vi "niFpgaScaledWinTemplate.vi"(0 "real data in":fxp<+/-,16,1>, 5 "imaginary data in":fxp<+/-,16,1>) -> (3 "data index":u16, 4 "real data out":fxp<+/-,18,2> format="%.17g", 6 "imaginary data out":fxp<+/-,18,2> format="%.17g")   [LabVIEW 2017]
uses:
  <vilib>/Platform/TimedLoop/XDataNode/timing_clust.ctl
  <vilib>/Platform/TimedLoop/XDataNode/nitl_modes.ctl
  <vilib>/Platform/TimedLoop/XDataNode/wakeup.ctl
  <vilib>/Platform/TimedLoop/XDataNode/XDataNode.xnode
  <vilib>/rvi/FXPMathLib/basic elements/FxpDiscreteDelay/XNode/nifxpmath_DiscreteDelay.xnode
  <vilib>/rvi/FXPMathLib/FxpMul/XNode/nifxpmath_Multiplier.xnode
  <vilib>/Platform/TimedLoop/XDataNode/XDNodeRunTimeDep.lvlib
  <vilib>/rvi/FXPMathLib/sim/FxpSim.dll
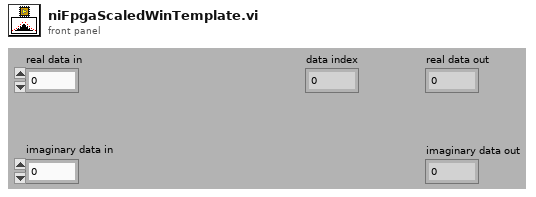
[diagram p1: front panel]
types:
  T1 = typedef "XDNodeRunTimeDep.lvlib/timing_clust.ctl" = cluster{"Expected End [f-1]":u64, "Actual End [f-1]":u64, "Finished Late? [f-1]":bool, "Expected End [i-1]":u64, "Actual End [i-1]":u64, "Finished Late? [i-1]":bool, "Expected Start [i]":u64, "Actual Start [i]":u64, "Expected Start [f]":u64, "Actual Start [f]":u64, "Source Name":string, "Structure Name":string, "Period":i64, "Deadline":i64, "Offset":i64, "Start":i64, "Priority":i32, "Timeout":i32, "Mode":T2, "Wakeup Reason":T3, "Error":errorcluster, "Source Type":string, "Secondary Source Type":string, "Global End Time":u64, "Global Start Time":u64, "Frame Duration":u64, "Iteration Duration":u64, "Assigned CPU":i32, "I/O Scan Engine Mode":u32}
  T2 = typedef "XDNodeRunTimeDep.lvlib/nitl_modes.ctl" = enum32{"No Change", "Process missed periods, maintain original phase", "Discard missed periods, maintain original phase", "Process missed periods, ignore original phase", "Discard missed periods, ignore original phase"}
  T3 = typedef "XDNodeRunTimeDep.lvlib/wakeup.ctl" = enum32{"Normal", "Aborted", "Asynchronous wakeup", "Timing source error", "Timed loop error", "Timeout"}
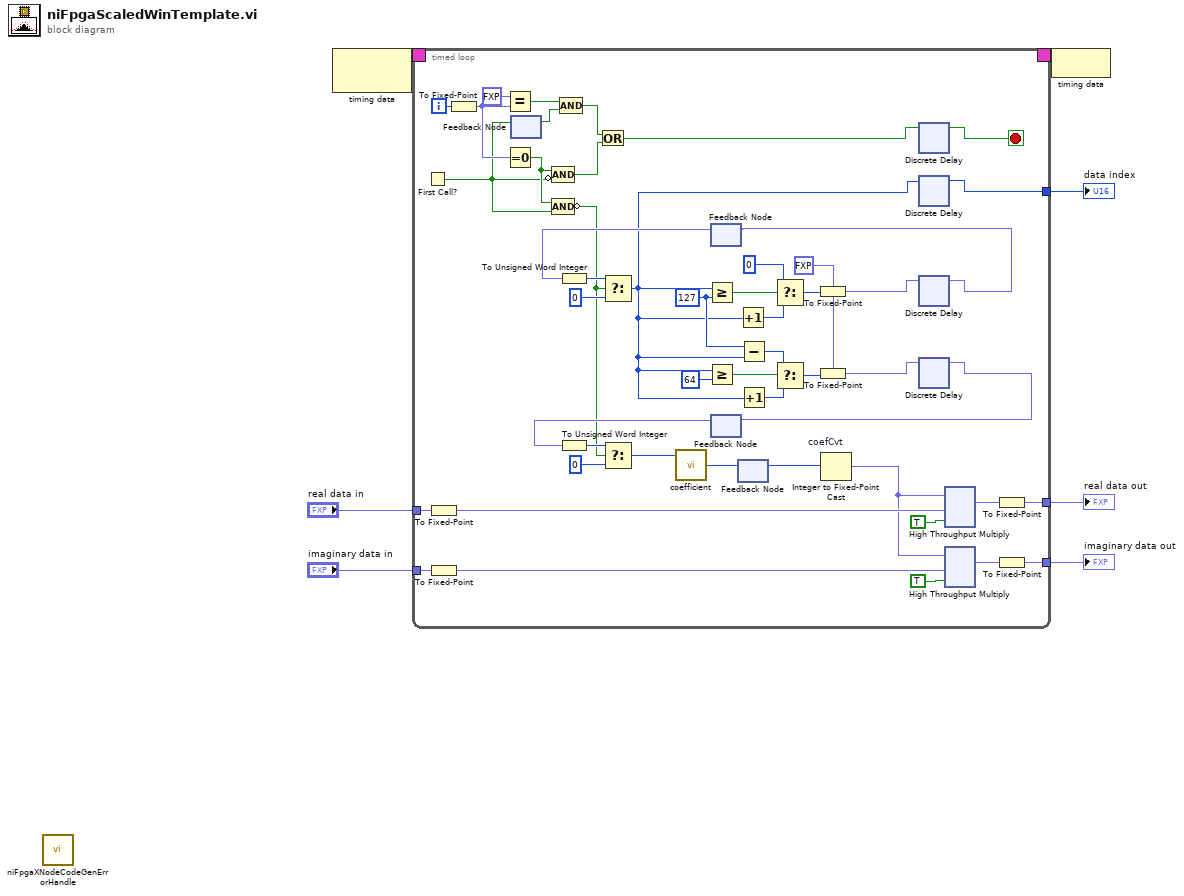
[diagram p0: block diagram]
diagram:
  n1 = call <vilib>:"niFpgaXNodeCodeGenErrorHandle.vi"() -> ()  [unwired: 1 in]
  n2 = node-c288() -> (w7:T1)  [unwired: 1 out]
  n3 = timed-loop "MainLoop" {
    tunnel: "real data in" -> [w36]
    tunnel: [w35] -> w2
    tunnel: "imaginary data in" -> [w13]
    tunnel: [w34] -> w1
    tunnel: [w32] -> w3
    timing: w7 -> [_]
    timing-out: [_] -> w6
    i -> [w52]
    stop <- w17 stop-if-true
    w44 = fxp<+,7,7> 0.0 ("LBitMask")
    w48 = u16 127 ("L-1")
    n4 = First Call?() -> (First Call?: T/F=w21:bool)
    n5 = To Fixed-Point(number=w36) -> (fixed-point=w14:fxp<+/-,16,1>)  [unwired: 1 in]
    n6 = To Fixed-Point(number=w13) -> (fixed-point=w12:fxp<+/-,16,1>)  [unwired: 1 in]
    n7 = To Fixed-Point(number=w52) -> (fixed-point=w22:fxp<+,3,3>)  [unwired: 1 out]
    n8 = Equal?(x=fxp<+,3,3> 1.0, y=w22) -> (x = y?=w24:bool)
    n9 = Equal To 0?(x=w22) -> (x = 0?=w27:bool)
    n10 = feedback-in #1(w21) -> ()
    n11 = feedback #1() -> (w25:bool)  [unwired: 1 out]
    n12 = Compound Arithmetic op=AND(w27, invert w21) -> (w26:bool)
    n13 = Compound Arithmetic op=AND(w27, w21) -> (invert w20:bool)
    n14 = Compound Arithmetic op=AND(w24, w25) -> (w15:bool)
    n15 = Or(x=w15, y=w26) -> (x .or. y?=w18:bool)
    n16 = feedback #2() -> (w38:fxp<+,7,7>)  [unwired: 1 in]
    n17 = To Unsigned Word Integer(number=w38) -> (unsigned 16bit integer=w40:u16)
    n18 = Select(t=w40, s=w20, f=u16 0) -> (s? t:f=w16:u16)
    n19 = Greater Or Equal?(x=w16, y=w48) -> (x >= y?=w53:bool)
    n20 = Greater Or Equal?(x=w16, y=u16 64 ("L/2")) -> (x >= y?=w54:bool)
    n21 = feedback #3() -> (w37:fxp<+,7,7>)  [unwired: 1 in]
    n22 = To Unsigned Word Integer(number=w37) -> (unsigned 16bit integer=w43:u16)
    n23 = Select(t=w43, s=w20, f=u16 0) -> (s? t:f=w45:u16)
    n24 = call "coefficient"("address"=w45) -> ("data out"=w39:i32)  [unwired: 8 in]
    n25 = Increment(x=w16) -> (x+1=w55:u16)
    n26 = feedback-in #4(w39) -> ()
    n27 = feedback #4() -> (w8:i32)  [unwired: 1 out]
    n28 = Subtract(x=w48, y=w16) -> (x-y=w50:u16)
    n29 = Increment(x=w16) -> (x+1=w49:u16)
    n30 = Select(t=u16 0, s=w53, f=w55) -> (s? t:f=w47:u16)
    n31 = Select(t=w50, s=w54, f=w49) -> (s? t:f=w46:u16)
    n32 = To Fixed-Point(fixed-point type=w44, number=w47) -> (fixed-point=w31:fxp<+,7,7>)
    n33 = To Fixed-Point(fixed-point type=w44, number=w46) -> (fixed-point=w29:fxp<+,7,7>)
    n34 = Integer to Fixed-Point Cast "coefCvt"(integer=w8) -> (fixed-point=w9:fxp<+/-,20,2>)  [unwired: 1 in]
    n35 = xnode "Discrete Delay"("D"=w18) -> ("Q"=w17:bool)
    n36 = xnode "Discrete Delay"("D"=w16) -> ("Q"=w32:u16)
    n37 = xnode "Discrete Delay"("D"=w31) -> ("Q"=w30:fxp<+,7,7>)
    n38 = feedback-in #2(w30) -> ()
    n39 = xnode "Discrete Delay"("D"=w29) -> ("Q"=w28:fxp<+,7,7>)
    n40 = feedback-in #3(w28) -> ()
    n41 = xnode "High Throughput Multiply"("x"=w9, "y"=w14, "input valid"=TRUE) -> ("x*y"=w19:fxp<+/-,36,3>)  [unwired: 1 in, 2 out]
    n42 = xnode "High Throughput Multiply"("x"=w9, "y"=w12, "input valid"=TRUE) -> ("x*y"=w33:fxp<+/-,36,3>)  [unwired: 1 in, 2 out]
    n43 = To Fixed-Point ("MultCast")(number=w19) -> (fixed-point=w35:fxp<+/-,18,2>)  [unwired: 1 out]
    n44 = To Fixed-Point ("MultCast")(number=w33) -> (fixed-point=w34:fxp<+/-,18,2>)  [unwired: 1 out]
  }
  "data index" <- w3
  "real data out" <- w2
  "imaginary data out" <- w1
  n45 = node-c288(w6) -> ()
